vi "Configure Frequency Burst Gate.vi"(6 "Gate Time (1E-6 s)":dbl=1e-06, 7 "Enable Narrow Pulse (F: Disable)":bool, 8 "error in (no error)":errorcluster, 9 "Delay Time (0 s)":dbl, 10 "Enable Auto Gate (T: Enable)":bool=TRUE, 11 "VISA resource name":refnum<visa-resource-name>) -> (0 "error out":errorcluster, 3 "VISA resource name out":refnum<visa-resource-name>)   [LabVIEW 2021, in "Agilent 532XX Series.lvlib"]
doc: "Configures the characteristics of frequency burst gate.\n\n<B>Note:</B> This VI only applies to the Agilent 53220A/53230A."
uses:
  <instrlib>/Agilent 532XX Series/Agilent 532XX Series.lvlib
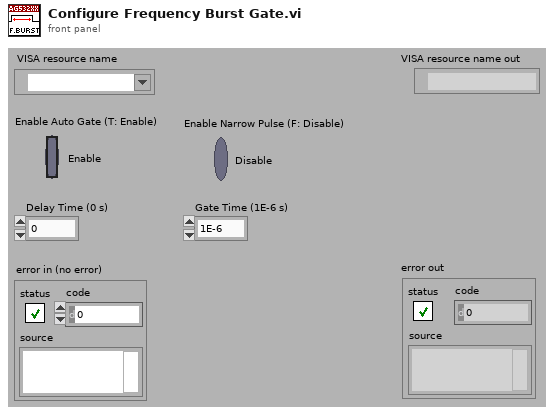
[diagram p1: front panel]
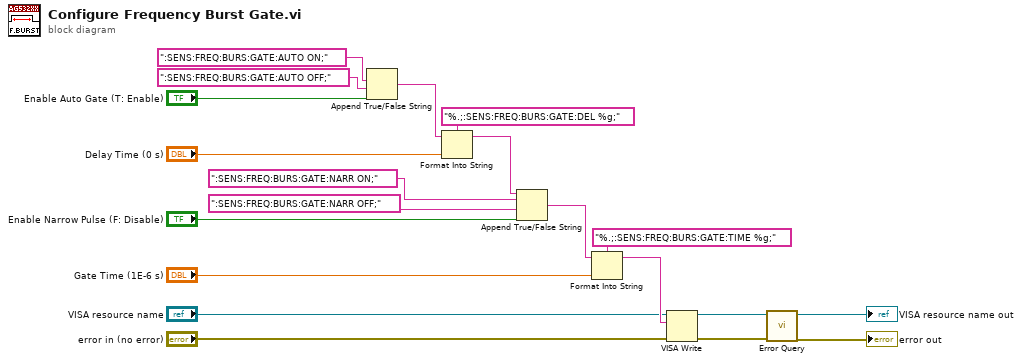
[diagram p0: block diagram]
diagram:
  n1 = Append True/False String(1:"Enable Auto Gate (T: Enable)", 2:":SENS:FREQ:BURS:GATE:AUTO OFF;", 3:":SENS:FREQ:BURS:GATE:AUTO ON;") -> (0:w17:string)  [unwired: 1 out]
  n2 = Format Into String(format string="%.;:SENS:FREQ:BURS:GATE:DEL %g;", initial string=w17, "Delay Time (0 s)") -> (resulting string=w14:string)  [unwired: 1 in, 1 out]
  n3 = Append True/False String(1:"Enable Narrow Pulse (F: Disable)", 2:":SENS:FREQ:BURS:GATE:NARR OFF;", 3:":SENS:FREQ:BURS:GATE:NARR ON;", 4:w14) -> (0:w10:string)
  n4 = Format Into String(format string="%.;:SENS:FREQ:BURS:GATE:TIME %g;", initial string=w10, "Gate Time (1E-6 s)") -> (resulting string=w7:string)  [unwired: 1 in, 1 out]
  n5 = VISA Write(VISA resource name="VISA resource name", write buffer=w7, error in (no error)="error in (no error)") -> (VISA resource name out=w4:refnum<visa-resource-name>, error out=w3:errorcluster)  [unwired: 1 out]
  n6 = call <instrlib>:"Error Query.vi"("error in (no error)"=w3, "VISA resource name"=w4) -> ("error out"=→"error out":errorcluster, "VISA resource name out"=→"VISA resource name out":refnum<visa-resource-name>)  [unwired: 8 out]
